vi "DM Get burst list.vi"(8 "error in (no error)":errorcluster, 11 "burst group":string) -> (0 "error out":errorcluster, 3 "burst info":T1)   [LabVIEW 2019, in "DataManagment.lvlib"]
uses:
  DataManagment.lvlib
  DM group info.ctl
  bf58cb7d-6bb3-4df0-820e-10d90c888869.vi
  bf58cb7d-6bb3-4df0-820e-10d90c888869.vi/f97d655a-a229-4f02-b13f-ff29dae763c6.vi
  bf58cb7d-6bb3-4df0-820e-10d90c888869.vi/bcbbce96-e988-4c70-97d9-37a38b06dc61.vi
  <vilib>/Utility/High Resolution Relative Seconds.vi
  <vilib>/Utility/error.llb/Clear Errors.vi
  <vilib>/addons/_JKI.lib/Serialization/JSON/Library/Unflatten From JSON String.vi
  <vilib>/addons/_JKI.lib/Serialization/JSON/JKI JSON Serialization.lvlib
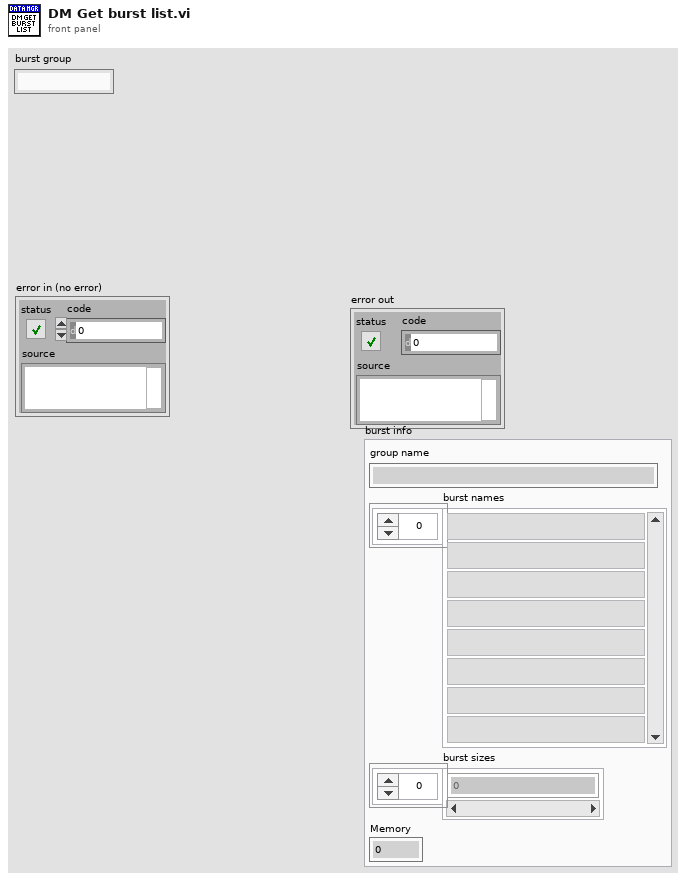
[diagram p1: front panel]
types:
  T1 = typedef "DataManagment.lvlib/DM group info.ctl" = cluster{"group name":string, "burst names":string[], "burst sizes":dbl[], "Memory":dbl}
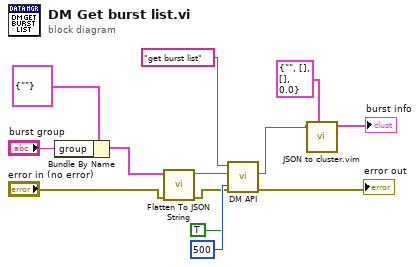
[diagram p0: block diagram]
diagram:
  n1 = Bundle By Name(cluster=cluster{"group":string} {"group"=""}, "group"="burst group") -> (w8:cluster{"group":string})
  n2 = call <vilib>:"Flatten To JSON String.vi"("error in (no error)"="error in (no error)", "Variant"=w8) -> ("error out"=w4:errorcluster, "JSON String"=w6:string)  [unwired: 8 in]
  n3 = call "DM API.vi"("response timeout(500)"=500, "response"=TRUE, "error in (no error)"=w4, "parameters"=w6, "message"="get burst list") -> ("error out"=→"error out":errorcluster, "response"=w2:string)  [unwired: 3 in, 2 out]
  n4 = call "JSON to cluster.vim"("data"=T1 {"group name"="", "burst names"=[], "burst sizes"=[], "Memory"=0.0} ("group info"), "JSON in"=w2) -> ("data"=→"burst info":T1)  [unwired: 7 in, 2 out]
